vi "Phase to Position.vi"(10 "Phase":dbl, 11 "Total Angle":dbl) -> (3 "x,y":dbl[](array[numeric]))   [LabVIEW 2021]
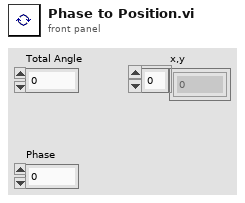
[diagram p1: front panel]
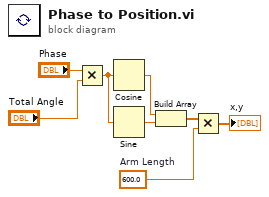
[diagram p0: block diagram]
diagram:
  w3 = 600.0  # Arm Length
  n1 = Multiply(x="Phase", y="Total Angle") -> (x*y=w7:dbl)
  n2 = Cosine(x=w7) -> (cos(x)=w1:dbl)
  n3 = Sine(x=w7) -> (sin(x)=w2:dbl)
  n4 = Build Array(w1, w2) -> (w4:dbl[])
  n5 = Multiply(x=w4, y=w3) -> (x*y=→"x,y":dbl[])
